vi "Create File Name.vi"(8 "error in (no error)":errorcluster, 11 "HIJ Vision Camera App in":refnum<class "HIJ Vision Camera App.lvclass">) -> (0 "error out":errorcluster, 2 "FileName":string, 3 "HIJ Vision Camera App out":refnum<class "HIJ Vision Camera App.lvclass">)   [LabVIEW 2020, in "HIJ Vision Camera App.lvlib" / "HIJ Vision Camera App.lvclass"]
uses:
  HIJ Vision Camera App.lvclass
  C:/Users/AlexK/work/LabVIEW Programme/POLARIS CAM Log Abw und E/Submodules/HIJ Vision/Application Base Actors/HIJ Vision Application/HIJ Vision Application/HIJ Vision Application.lvclass
  HIJ Vision Camera App.lvclass/HIJ Vision Camera App.ctl
  HIJ Vision Application/HIJ Vision Application/HIJ Vision Application.lvclass/HIJ Vision Application.ctl
  Read Prefix.vi
  Read Camera Name.vi
  Read Save Source in Filename.vi
  Read ShotIdInFileName.vi
  HIJ Vision Application/HIJ Vision Application/Read ShotID.vi
  Read FrameNrInFilename.vi
  Read Frame Nr.vi
  Read TimestampFormat.vi
  Read ImageTimeStamp.vi
  Read SaveTimestamp.vi
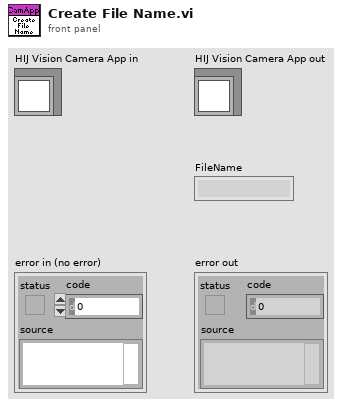
[diagram p1: front panel]
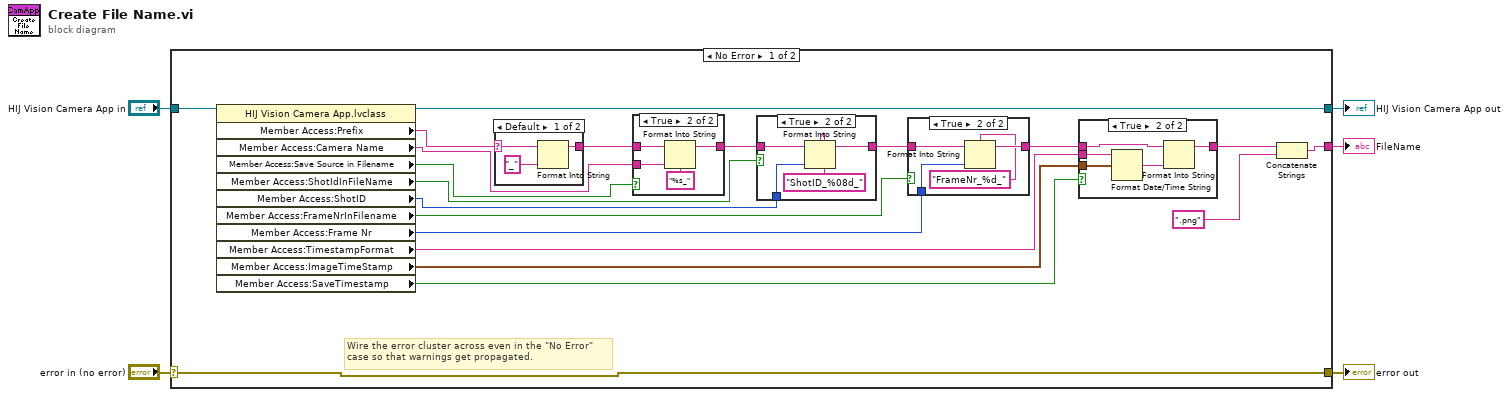
[diagram p0: block diagram]
diagram:
  n1 = case shown="No Error" "error in (no error)" {
    selector: "error in (no error)" -> [w25 w52]
    tunnel: [w25 w52] -> w4
    tunnel: [w10 w51] -> w2
    tunnel: "HIJ Vision Camera App in" -> [w9 w51]
    tunnel: [w7 _] -> w1
    frame No Error {
      # "Wire the error cluster across even in the \"No Error\"\ncase so that warnings get propagated."
      n2 = property class="HIJ Vision Camera App.lvclass"(reference=w9) -> (reference out=w10:refnum<class "HIJ Vision Camera App.lvclass">, "Member Access:Prefix"=w21:string, "Member Access:Camera Name"=w22:string, "Member Access:Save Source in Filename"=w23:bool, "Member Access:ShotIdInFileName"=w15:bool, "Member Access:ShotID"=w16:i32, "Member Access:FrameNrInFilename"=w19:bool, "Member Access:Frame Nr"=w18:i32, "Member Access:TimestampFormat"=w11:string, "Member Access:ImageTimeStamp"=w13:timestamp, "Member Access:SaveTimestamp"=w12:bool)  [unwired: 1 in, 1 out]
      n3 = case shown="Default" w21 {
        selector: w21 -> [w28 w29]
        tunnel: [w27 w29] -> w24
        frame Default {
          n4 = Format Into String(initial string=w28, "_") -> (resulting string=w27:string)  [unwired: 2 in, 1 out]
        }
        frame "" {
        }
      }
      n5 = case shown="True" w23 {
        tunnel: [w30 w34] -> w20
        tunnel: w24 -> [w30 w33]
        tunnel: w22 -> [_ w32]
        frame False {
        }
        frame True {
          n6 = Format Into String(format string="%s_", initial string=w33, w32) -> (resulting string=w34:string)  [unwired: 1 in, 1 out]
        }
      }
      n7 = case shown="True" w15 {
        tunnel: w20 -> [w35 w39]
        tunnel: [w35 w38] -> w14
        tunnel: w16 -> [_ w37]
        frame False {
        }
        frame True {
          n8 = Format Into String(format string="ShotID_%08d_", initial string=w39, w37) -> (resulting string=w38:string)  [unwired: 1 in, 1 out]
        }
      }
      n9 = case shown="True" w19 {
        tunnel: w14 -> [w40 w44]
        tunnel: [w40 w43] -> w17
        tunnel: w18 -> [_ w41]
        frame False {
        }
        frame True {
          n10 = Format Into String(format string="FrameNr_%d_", initial string=w44, w41) -> (resulting string=w43:string)  [unwired: 1 in, 1 out]
        }
      }
      n11 = case shown="True" w12 {
        tunnel: [w45 w46] -> w8
        tunnel: w17 -> [w45 w48]
        tunnel: w11 -> [_ w50]
        tunnel: w13 -> [_ w47]
        frame False {
        }
        frame True {
          n12 = Format Date/Time String(time format string (%c)=w50, seconds (now)=w47) -> (date/time string=w49:string)  [unwired: 1 in]
          n13 = Format Into String(initial string=w48, w49) -> (resulting string=w46:string)  [unwired: 2 in, 1 out]
        }
      }
      n14 = Concatenate Strings(w8, ".png" ("string")) -> (w7:string)
    }
    frame Error {
    }
  }
  "error out" <- w4
  "HIJ Vision Camera App out" <- w2
  "FileName" <- w1
